vi "Test synchronisation.vi"   [LabVIEW 2020]
uses:
  synchronization/synchronization.lvclass
  <vilib>/numeric/Random Number (Range) U64.vi
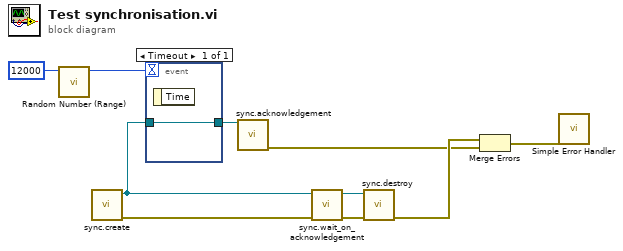
[diagram p0: block diagram]
diagram:
  n1 = call-poly <vilib>:"Random Number (Range).vi"("upper bound (100)"=u64 12000) -> ("number"=w7:u64)  [unwired: 10 in]
  n2 = call "sync.create.vi"() -> ("error out"=w8:errorcluster, "synchronization"=w5:refnum<class "synchronization.lvclass">)  [unwired: 10 in]
  n3 = event shown="[0] Timeout" {
    selector: _ -> [_]
    dyn-events: _ -> [_]
    timeout: w7 -> [_]
    tunnel: w5 -> [w11]
    tunnel: [w11] -> w4
    event Timeout {
      n4 = event-data() -> ()  [unwired: 1 in, 1 out]
    }
  }
  n5 = call "sync.acknowledgement.vi"("synchronization"=w4) -> ("error out"=w2:errorcluster)  [unwired: 9 in, 1 out]
  n6 = call "sync.wait_on_acknowledgement.vi"("error in (no error)"=w8, "synchronization in"=w5) -> ("error out"=w9:errorcluster, "synchronization out"=w10:refnum<class "synchronization.lvclass">)  [unwired: 8 in]
  n7 = call "sync.destroy.vi"("error in (no error)"=w9, "synchronization"=w10) -> ("error out"=w3:errorcluster)  [unwired: 9 in]
  n8 = Merge Errors(w3, w2) -> (w1:errorcluster)
  n9 = call <vilib>:"Simple Error Handler.vi"("error in (no error)"=w1) -> ()  [unwired: 4 in, 5 out]
